vi "Plot load - general.vi"(7 "First call? (init)":bool, 8 "error in (no error)":errorcluster, 10 "General":T1={"Title"="", "Time to Plot"=1800.0, "Title.Visible"=FALSE, "Sidebar.Visible"=FALSE, "Plot Area:Colors:BG Color"=0, "X Scale.Plot Name"="", "X Scale.Use Plot Name"=FALSE} {"Time to Plot" format="%<%M:%S>t"}, 11 "Refs":T2) -> (0 "error out":errorcluster)   [LabVIEW 2021, in "RocketPlot.lvlib"]
uses:
  RocketPlot.lvlib
  TypeDefs/Plot UI references.ctl
  Classes/RocketPlotHandle/RocketPlotHandle.lvclass
  <userlib>/bjustice/TipStripOOPanel/Classes/TipPanelHandle/TipPanelHandle.lvclass
  TypeDefs/Plot top row.ctl
  TypeDefs/Plot general properties.ctl
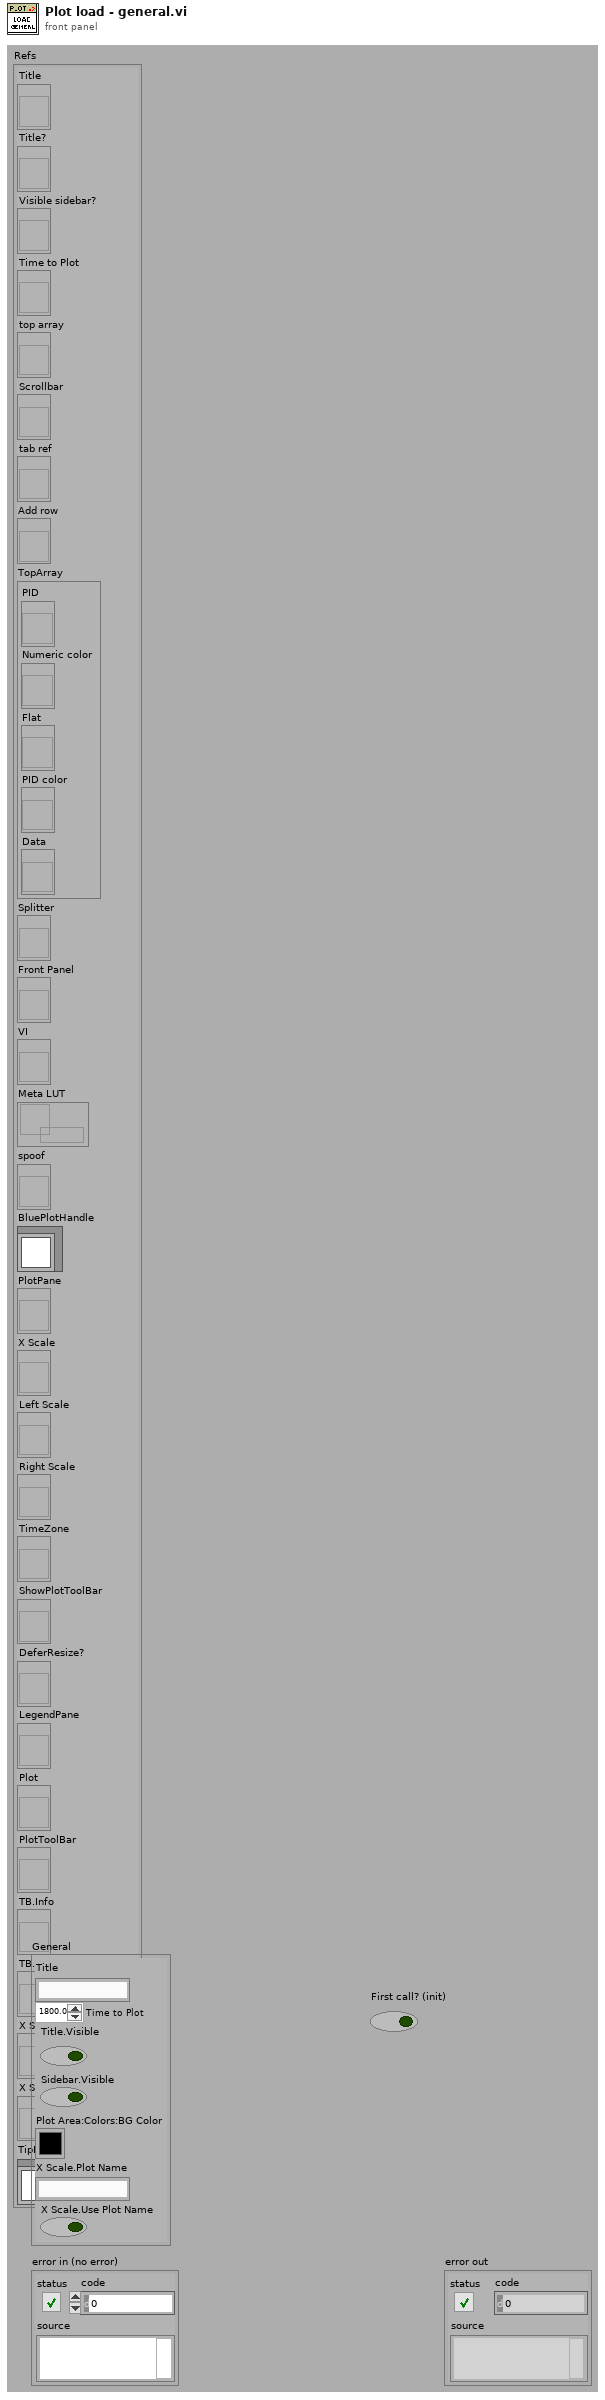
[diagram p1: front panel]
types:
  T1 = typedef "RocketPlot.lvlib/Plot general properties.ctl" = cluster{"Title":string, "Time to Plot":dbl, "Title.Visible":bool, "Sidebar.Visible":bool, "Plot Area:Colors:BG Color":u32, "X Scale.Plot Name":string, "X Scale.Use Plot Name":bool}
  T2 = typedef "RocketPlot.lvlib/Plot UI references.ctl" = cluster{"Title":refnum<vi>, "Title?":refnum<vi>, "Visible sidebar?":refnum<vi>, "Time to Plot":refnum<vi>, "top array":refnum<vi>, "Scrollbar":refnum<vi>, "tab ref":refnum<vi>, "Add row":refnum<vi>, "TopArray":cluster{"PID":refnum<vi>, "Numeric color":refnum<vi>, "Flat":refnum<vi>, "PID color":refnum<vi>, "Data":refnum<vi>}, "Splitter":refnum<vi>, "Front Panel":refnum<vi>, "VI":refnum<vi>, "Meta LUT":refnum<data-value>, "spoof":refnum<vi>, "BluePlotHandle":refnum<class "RocketPlotHandle.lvclass">, "PlotPane":refnum<vi>, "X Scale":refnum<vi>, "Left Scale":refnum<vi>, "Right Scale":refnum<vi>, "TimeZone":refnum<vi>, "ShowPlotToolBar":refnum<vi>, "DeferResize?":refnum<vi>, "LegendPane":refnum<vi>, "Plot":refnum<vi>, "PlotToolBar":refnum<vi>, "TB.Info":refnum<vi>, "TB.max":refnum<vi>, "X Scale.Plot Name":refnum<vi>, "X Scale.Use Plot Name?":refnum<vi>, "TipPanel":refnum<class "TipPanelHandle.lvclass">}
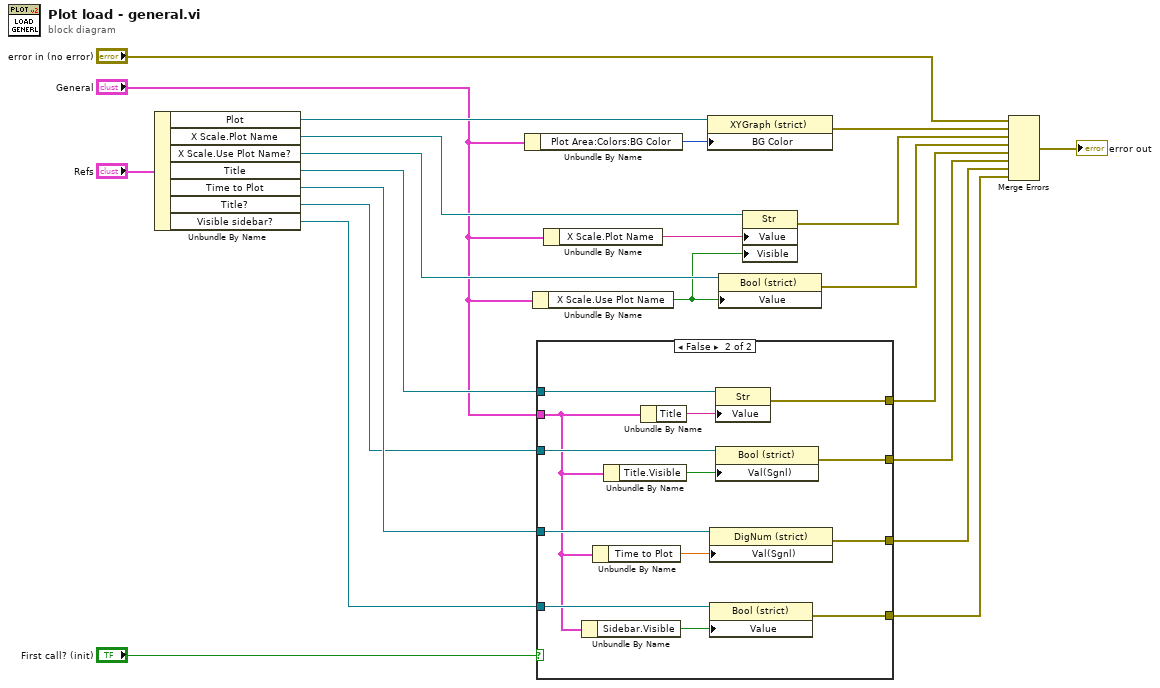
[diagram p0: block diagram]
diagram:
  n1 = Unbundle By Name("Refs") -> ("Plot"=w15:refnum<vi>, "X Scale.Plot Name"=w6:refnum<vi>, "X Scale.Use Plot Name?"=w5:refnum<vi>, "Title"=w14:refnum<vi>, "Time to Plot"=w19:refnum<vi>, "Title?"=w13:refnum<vi>, "Visible sidebar?"=w22:refnum<vi>)
  n2 = Unbundle By Name("General") -> ("Plot Area:Colors:BG Color"=w9:u32)
  n3 = Unbundle By Name("General") -> ("X Scale.Use Plot Name"=w1:bool)
  n4 = case shown="False" "First call? (init)" {
    tunnel: w22 -> [_ w34]
    tunnel: "General" -> [_ w23]
    tunnel: [_ w33] -> w20
    tunnel: w19 -> [_ w31]
    tunnel: [_ w30] -> w18
    tunnel: w14 -> [_ w27]
    tunnel: w13 -> [_ w26]
    tunnel: [_ w25] -> w12
    tunnel: [_ w24] -> w11
    frame True {
      # "These things are handled\non init in main\nDon't override here."
    }
    frame False {
      n5 = Unbundle By Name(w23) -> ("Sidebar.Visible"=w35:bool)
      n6 = Unbundle By Name(w23) -> ("Time to Plot"=w32:dbl)
      n7 = Unbundle By Name(w23) -> ("Title.Visible"=w29:bool)
      n8 = Unbundle By Name(w23) -> ("Title"=w28:string)
      n9 = property class="DigNum (strict)"(reference=w31, "Val(Sgnl)"=w32) -> (error out=w30:errorcluster)  [unwired: 1 in, 1 out]
      n10 = property class="Bool (strict)"(reference=w34, "Value"=w35) -> (error out=w33:errorcluster)  [unwired: 1 in, 1 out]
      n11 = property class="Str"(reference=w27, "Value"=w28) -> (error out=w25:errorcluster)  [unwired: 1 in, 1 out]
      n12 = property class="Bool (strict)"(reference=w26, "Val(Sgnl)"=w29) -> (error out=w24:errorcluster)  [unwired: 1 in, 1 out]
    }
  }
  n13 = Unbundle By Name("General") -> ("X Scale.Plot Name"=w7:string)
  n14 = property class="XYGraph (strict)"(reference=w15, "BG Color"=w9) -> (error out=w21:errorcluster)  [unwired: 1 in, 1 out]
  n15 = property class="Bool (strict)"(reference=w5, "Value"=w1) -> (error out=w2:errorcluster)  [unwired: 1 in, 1 out]
  n16 = property class="Str"(reference=w6, "Value"=w7, "Visible"=w1) -> (error out=w3:errorcluster)  [unwired: 1 in, 1 out]
  n17 = Merge Errors("error in (no error)", w21, w3, w2, w12, w11, w18, w20) -> (→"error out":errorcluster)
